vi "S2C_VLFT10_Proc_RfPaths.vi"(8 "Error In":errorcluster, 11 "HandSwitch":string) -> (0 "Error Out":errorcluster, 3 "Result":string)   [LabVIEW 2015]
uses:
  Typedefs/S2C_VLFT10_Type_HandSwitch.ctl
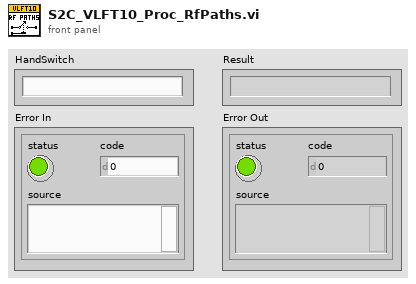
[diagram p1: front panel]
types:
  T1 = typedef "S2C_VLFT10_Type_HandSwitch.ctl" = u16
  T2 = cluster{"RF Path":T1, "Active?":bool, "DiffProbe?":bool}
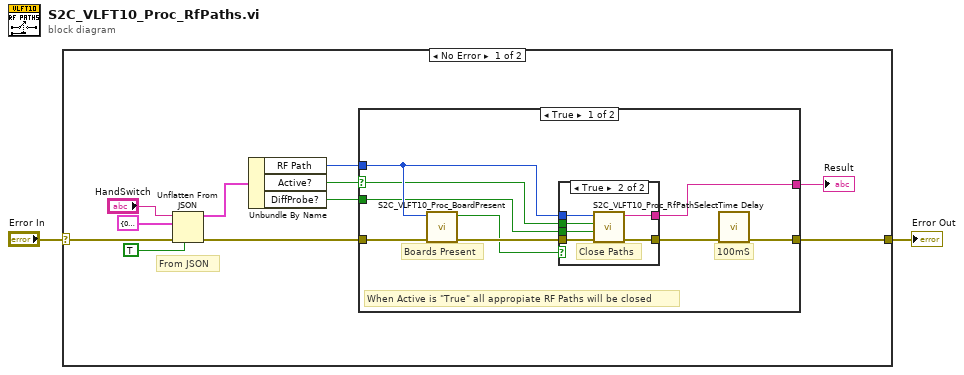
[diagram p0: block diagram]
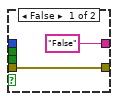
[diagram p2: hidden frame]
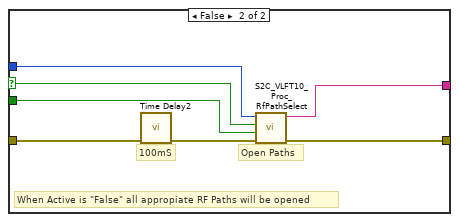
[diagram p3: hidden frame]
diagram:
  n1 = case shown="No Error" "Error In" {
    selector: "Error In" -> [w11 w38]
    tunnel: [w8 w38] -> w2
    frame No Error {
      # "From JSON"
      n2 = Unflatten From JSON(JSON string="HandSwitch", type and defaults=T2 {"RF Path"=0, "Active?"=FALSE, "DiffProbe?"=FALSE}, default null elements? (F)=TRUE, error in (no error)=w11) -> (value=w7:T2, error out=w10:errorcluster)  [unwired: 3 in]
      n3 = Unbundle By Name(w7) -> ("RF Path"=w6:T1, "Active?"=w4:bool, "DiffProbe?"=w5:bool)
      n4 = case shown="True" w4 {
        selector: w4 -> [w17 w32]
        tunnel: w10 -> [w22 w33]
        tunnel: [w15 w34] -> w9
        tunnel: [w16 w35] -> w8
        tunnel: w6 -> [w19 w36]
        tunnel: w5 -> [w18 w31]
        frame True {
          # "When Active is \"True\" all appropiate RF Paths will be closed"
          # "100mS"
          # "Boards Present"
          n5 = call "S2C_VLFT10_Proc_BoardPresent.vi"("Error In"=w22, "HandSwitch"=w19) -> ("Error Out"=w21:errorcluster, "Present?"=w14:bool)  [unwired: 8 in]
          n6 = case shown="True" w14 {
            tunnel: w21 -> [w24 w30]
            tunnel: w17 -> [_ w29]
            tunnel: w18 -> [_ w28]
            tunnel: w19 -> [_ w27]
            tunnel: ["False" ("Result") w26] -> w15
            tunnel: [w24 w25] -> w20
            frame False {
            }
            frame True {
              # "Close Paths"
              n7 = call "S2C_VLFT10_Proc_RfPathSelect.vi"("Error In"=w30, "DiffProbe?"=w28, "Active?"=w29, "HandSwitch"=w27) -> ("Error Out"=w25:errorcluster, "Result"=w26:string)  [unwired: 6 in]
            }
          }
          n8 = call "Time Delay"("error in (no error)"=w20) -> ("error out"=w16:errorcluster)  [unwired: 10 in]
        }
        frame False {
          # "When Active is \"False\" all appropiate RF Paths will be opened"
          # "Open Paths"
          # "100mS"
          n9 = call "Time Delay2"("error in (no error)"=w33) -> ("error out"=w37:errorcluster)  [unwired: 10 in]
          n10 = call "S2C_VLFT10_Proc_RfPathSelect.vi"("Error In"=w37, "DiffProbe?"=w31, "Active?"=w32, "HandSwitch"=w36) -> ("Error Out"=w35:errorcluster, "Result"=w34:string)  [unwired: 6 in]
        }
      }
      "Result" <- w9
    }
    frame Error {
    }
  }
  "Error Out" <- w2
